vi "wf_master.vi"(3 "format":string="%.6f", 4 "lower limit":dbl=-10.0, 5 "template":string="SOUR<channel>:VOLT:LOW <value>;", 6 "upper limit":dbl=10.0 format="%#_13g", 7 "override":bool, 8 "error in (no error)":errorcluster, 9 "options":string, 10 "value":dbl, 11 "VISA IN":refnum<visa-resource-name>) -> (0 "error out":errorcluster, 2 "value out":dbl=-3.829999999999993)   [LabVIEW 2017]
uses:
  <vilib>/Instr/_visa.llb/Select Event Type.ctl
  hardware/serial/serial.lvlib
panel:
  in  "VISA (default)":refnum<visa-resource-name>="33500B"
  out "cmds":string="SOUR1:VOLT:LOW -3.830000;"
  out "num_commands":i32=1 caption="num_cmds"
  in  "send":bool=TRUE
  # "options: channel or comma-delimited list of channels\nNB. limits and format string are usually overwritten by var_master.vi"
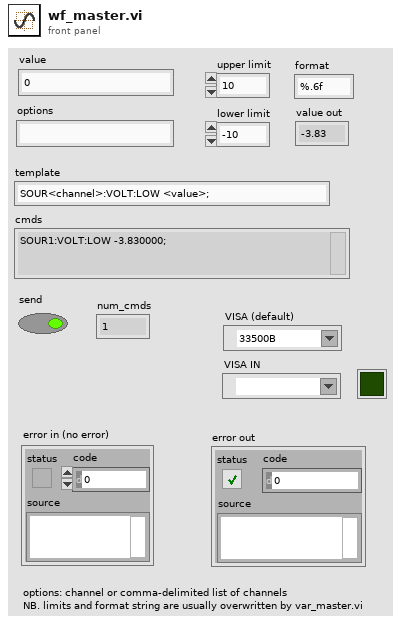
[diagram p1: front panel]
types:
  T1 = typedef "Select Event Type.ctl" = u32
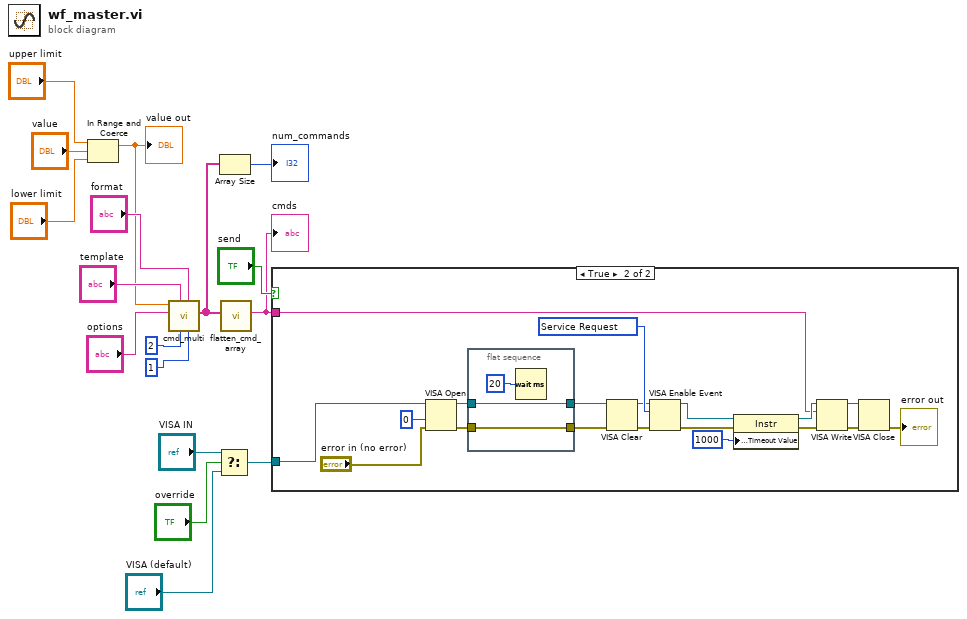
[diagram p0: block diagram]
diagram:
  n1 = In Range and Coerce(upper limit="upper limit", x="value", lower limit="lower limit") -> (coerced(x)=w12:dbl)  [unwired: 1 out]
  "value out" <- w12
  n2 = call "cmd_multi.vi"("chan_lower limit"=1, "value format"="format", "chan_upper limit"=2, "template"="template", "channel_list"="options", "value"=w12) -> ("cmds"=w8:string[])  [unwired: 4 in, 1 out]
  n3 = Select(t="VISA IN", s="override", f="VISA (default)") -> (s? t:f=w1:refnum<visa-resource-name>)
  n4 = Array Size(array=w8) -> (size(s)=→"num_commands":i32)
  n5 = call "flatten_cmd_array.vi"("cmd_array"=w8) -> ("cmds"=w7:string)  [unwired: 10 in]
  "cmds" <- w7
  n6 = case shown="True" "send" {
    tunnel: w7 -> [_ w19]
    tunnel: w1 -> [_ w18]
    frame False {
    }
    frame True {
      w27 = T1 1073684491 items=["Service Request"=1073684491, "Trigger"=3221168138, "Clear"=1073684493, "VXI Signal"=1073684512, "VXI/VME Interrupt"=3221168161, "VXI/VME Sysfail"=1073684509, "VXI/VME Sysreset"=1073684510, "GPIB CIC"=1073684498, "GPIB Talk"=1073684499, "GPIB Listen"=1073684500, "PXI Interrupt"=1073684514, "Serial Break"=1073684515, "Serial TermChar"=1073684516, "Serial CTS"=1073684521, "Serial DSR"=1073684522, "Serial DCD"=1073684524, "Serial RI"=1073684526, "Serial Character"=1073684533, "USB Interrupt"=1073684535, "All Enabled"=1073709055] ("Event Type")
      n7 = VISA Open(access mode=u32 0, error in (no error)="error in (no error)", VISA resource name=w18) -> (VISA resource name=w29:refnum<visa-resource-name>, error out=w31:errorcluster)  [unwired: 2 out]
      n8 = flat-sequence {
        tunnel: w31 -> [w39]
        tunnel: [w39] -> w30
        tunnel: w29 -> [w38]
        tunnel: [w38] -> w28
        frame #0 {
          n9 = Wait (ms)(milliseconds to wait=u32 20) -> ()  [unwired: 1 out]
        }
      }
      n10 = VISA Clear(VISA resource name=w28, error in (no error)=w30) -> (VISA resource name out=w26:refnum<visa-resource-name>, error out=w25:errorcluster)
      n11 = VISA Enable Event(8:w25, 10:w27, 11:w26) -> (0:w24:errorcluster, 3:w23:refnum<visa-resource-name>)  [unwired: 1 in]
      n12 = property class="Instr"(reference=w23, error in=w24, "General Settings:Timeout Value"=u32 1000) -> (reference out=w22:refnum<visa-resource-name>, error out=w32:errorcluster)
      n13 = VISA Write(VISA resource name=w22, write buffer=w19, error in (no error)=w32) -> (VISA resource name out=w20:refnum<visa-resource-name>, error out=w21:errorcluster)  [unwired: 1 out]
      n14 = VISA Close(VISA resource name=w20, error in (no error)=w21) -> (error out=→"error out":errorcluster)
    }
  }
